vi "Handle Error.vi"(8 "error in (no error)":errorcluster, 11 "Target Reply Time Test Actor in":refnum<class "Target Reply Time Test Actor.lvclass">) -> (0 "error out":errorcluster, 2 "stop actor?":bool=TRUE, 3 "Target Reply Time Test Actor out":refnum<class "Target Reply Time Test Actor.lvclass">)   [LabVIEW 2023, in "Target Reply Time Test Actor.lvlib" / "Target Reply Time Test Actor.lvclass"]
doc: "(<B>Filename</B>: Actor Framework.lvlib:Actor.lvclass:Handle Error.vi)\n\nDefines how the actor handles an error that occurred while processing a message. By default, this method does nothing except stop the actor."
uses:
  Target Reply Time Test Actor.lvclass
  Target Reply Time Test Actor.lvclass/Target Reply Time Test Actor.ctl
  <vilib>/ActorFramework/Actor/Actor.lvclass
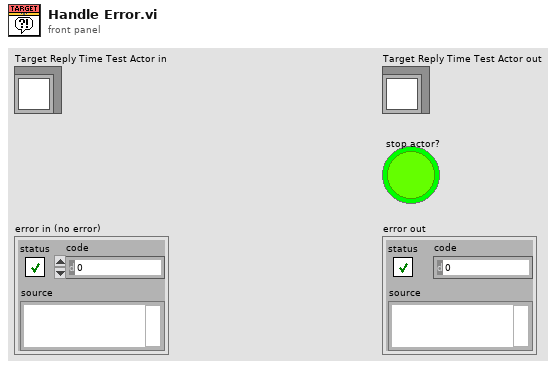
[diagram p1: front panel]
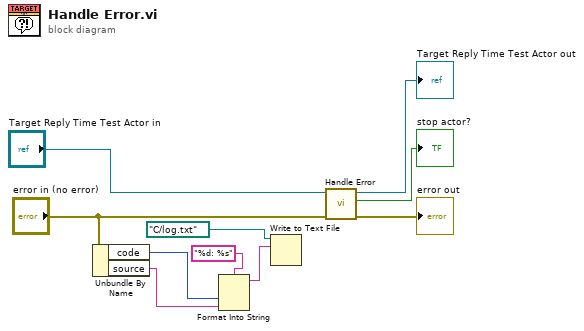
[diagram p0: block diagram]
diagram:
  n1 = Unbundle By Name("error in (no error)") -> ("code"=w4:i32, "source"=w1:string)
  n2 = Format Into String(format string="%d: %s", w4, w1) -> (resulting string=w3:string)  [unwired: 2 in, 1 out]
  n3 = Write to Text File(file (use dialog)=path "C:/log.txt", text=w3) -> ()  [unwired: 2 in, 3 out]
  n4 = call-parent "Handle Error.vi"("error in (no error)"="error in (no error)", "Actor in"="Target Reply Time Test Actor in") -> ("error out"=→"error out":errorcluster, "stop actor?"=→"stop actor?":bool, "Actor out"=→"Target Reply Time Test Actor out":refnum<class "Target Reply Time Test Actor.lvclass">)  [unwired: 7 in]
